vi "cost_evaluation.vi"(8 "Error In":errorcluster, 11 "GenAlg_data":T1) -> (0 "Error Out":errorcluster, 3 "GenAlg_data-out":T1)   [LabVIEW 2016]
uses:
  TypeDefs/GenAlg_data.ctl
  TypeDefs/basic_config.ctl
  TypeDefs/element.ctl
  TypeDefs/geration_data.ctl
  TypeDefs/selection_data.ctl
  TypeDefs/SimulatedAnnealing_data.ctl
  TypeDefs/multi_eval_data.ctl
  TypeDefs/termination_data.ctl
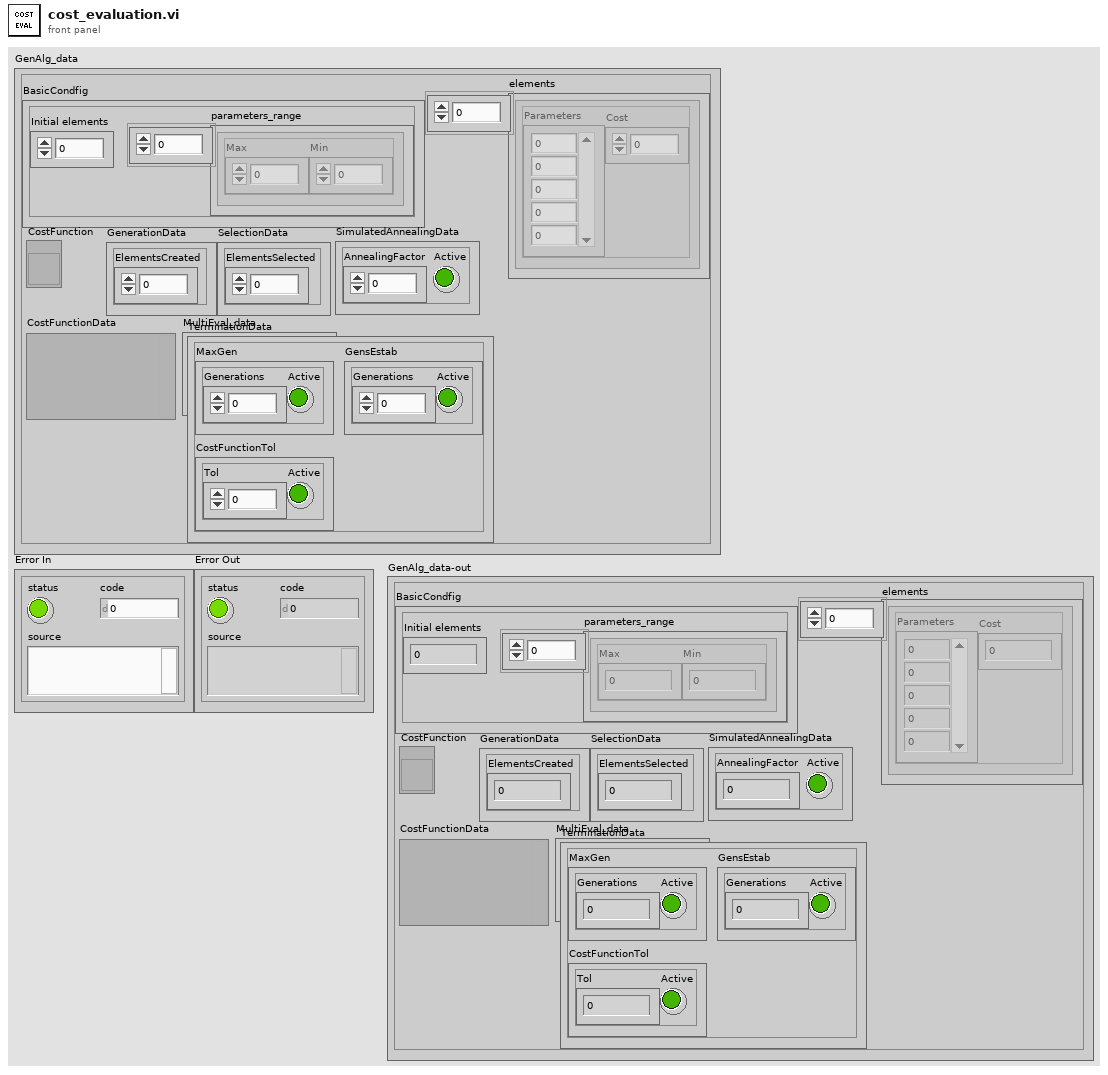
[diagram p1: front panel]
types:
  T1 = typedef "GenAlg_data.ctl" = cluster{"BasicCondfig":T2, "elements":T3[], "CostFunction":refnum<vi>, "GenerationData":T4, "SelectionData":T5, "SimulatedAnnealingData":T6, "CostFunctionData":variant, "MultiEval_data":T7, "TerminationData":T8}
  T2 = typedef "basic_config.ctl" = cluster{"parameters_range":cluster{"Max":dbl, "Min":dbl}[], "Initial elements":i32}
  T3 = typedef "element.ctl" = cluster{"Parameters":dbl[], "Cost":dbl}
  T4 = typedef "geration_data.ctl" = cluster{"ElementsCreated":i32}
  T5 = typedef "selection_data.ctl" = cluster{"ElementsSelected":i32}
  T6 = typedef "SimulatedAnnealing_data.ctl" = cluster{"AnnealingFactor":dbl, "Active":bool}
  T7 = typedef "multi_eval_data.ctl" = cluster{"Active":bool, "MultiEvalFunction":refnum<vi>}
  T8 = typedef "termination_data.ctl" = cluster{"MaxGen":cluster{"Generations":i32, "Active":bool}, "CostFunctionTol":cluster{"Tol":dbl, "Active":bool}, "GensEstab":cluster{"Generations":i32, "Active":bool}}
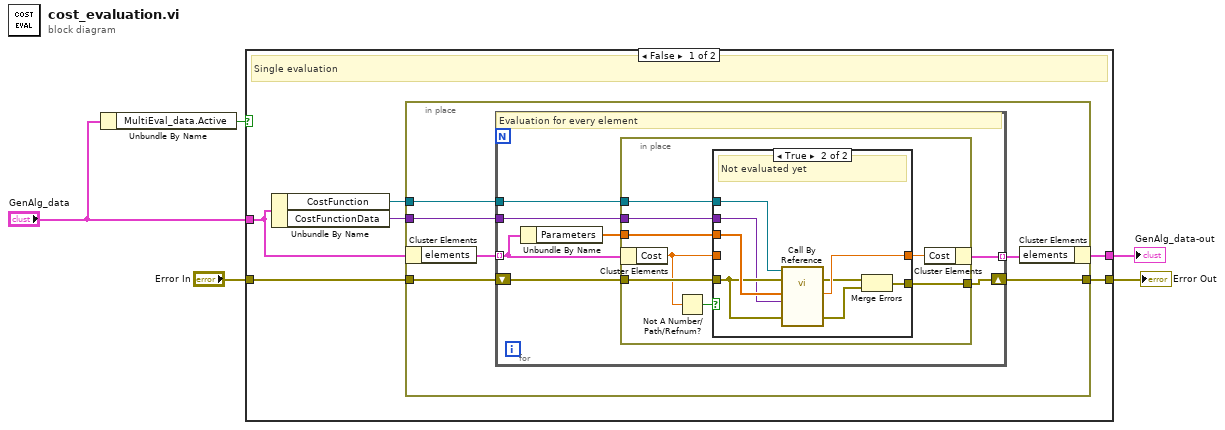
[diagram p0: block diagram]
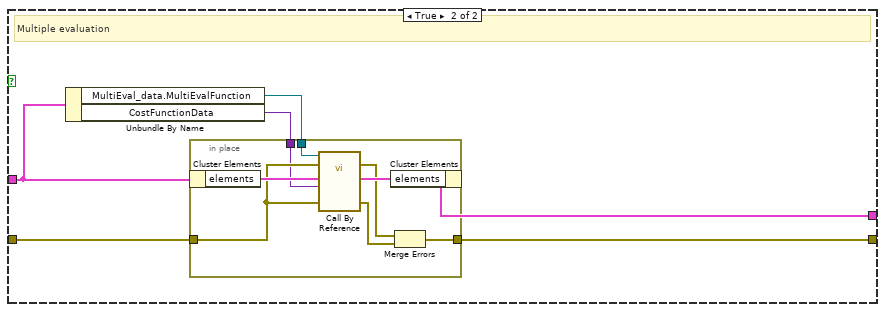
[diagram p3: hidden frame]
diagram:
  n1 = Unbundle By Name("GenAlg_data") -> ("MultiEval_data.Active"=w1:bool)
  n2 = case shown="False" w1 {
    tunnel: "Error In" -> [w10 w46]
    tunnel: [w9 w45] -> w4
    tunnel: [w8 w44] -> w3
    tunnel: "GenAlg_data" -> [w7 w48]
    frame False {
      # "Single evaluation"
      n3 = Unbundle By Name(w7) -> ("CostFunction"=w6:refnum<vi>, "CostFunctionData"=w11:variant)
      n4 = in-place {
        in-place-border: w11 -> [w17]
        in-place-border: w10 -> [w16]
        in-place-border: [w13] -> w9
        in-place-border: w6 -> [w12]
        n5 = in-place-cluster #1(w7) -> ("elements"=w15:T3[])
        n6 = for {
          tunnel: w15 -> [w20] mode=indexing
          tunnel: w17 -> [w24]
          shift-right: [w22] -> w13
          shift-left: w16 -> [w23]
          tunnel: [w21] -> w14 mode=indexing
          tunnel: w12 -> [w18]
          # "Evaluation for every element"
          n7 = Unbundle By Name(w20) -> ("Parameters"=w19:dbl[])
          n8 = in-place {
            in-place-border: w24 -> [w32]
            in-place-border: w23 -> [w31]
            in-place-border: [w29] -> w22
            in-place-border: w19 -> [w27]
            in-place-border: w18 -> [w25]
            n9 = in-place-cluster #2(w20) -> ("Cost"=w26:dbl)
            n10 = Not A Number/Path/Refnum?(number/path/refnum=w26) -> (NaN/Path/Refnum?=w28:bool)
            n11 = case shown="True" w28 {
              tunnel: w32 -> [_ w35]
              tunnel: w27 -> [_ w42]
              tunnel: w31 -> [w33 w41]
              tunnel: [w34 w40] -> w30
              tunnel: [w33 w37] -> w29
              tunnel: w26 -> [w34 _]
              tunnel: w25 -> [_ w36]
              frame False {
              }
              frame True {
                # "Not evaluated yet"
                n12 = call-by-ref "?"(reference=w36, error in=w41, "Error In"=w41, "Data"=w35, "Parameters"=w42) -> (error out=w38:errorcluster, "Error Out"=w39:errorcluster, "Cost"=w40:dbl)  [unwired: 7 in, 1 out]
                n13 = Merge Errors(w38, w39) -> (w37:errorcluster)
              }
            }
            n14 = in-place-cluster #2("Cost"=w30) -> (w21:T3)
          }
        }
        n15 = in-place-cluster #1("elements"=w14) -> (w8:T1)
      }
    }
    frame True {
      # "Multiple evaluation"
      n16 = Unbundle By Name(w48) -> ("MultiEval_data.MultiEvalFunction"=w47:refnum<vi>, "CostFunctionData"=w43:variant)
      n17 = in-place {
        in-place-border: w47 -> [w56]
        in-place-border: w46 -> [w53]
        in-place-border: [w50] -> w45
        in-place-border: w43 -> [w49]
        n18 = in-place-cluster #3(w48) -> ("elements"=w55:T3[])
        n19 = call-by-ref "?"(reference=w56, error in=w53, "Error In"=w53, "Data"=w49, "Elements"=w55) -> (error out=w51:errorcluster, "Error Out"=w52:errorcluster, "Elements out"=w54:T3[])  [unwired: 7 in, 1 out]
        n20 = in-place-cluster #3("elements"=w54) -> (w44:T1)
        n21 = Merge Errors(w51, w52) -> (w50:errorcluster)
      }
    }
  }
  "Error Out" <- w4
  "GenAlg_data-out" <- w3
